vi "Dialog - Configure Packet Header.vi"(8 "error in (no error)":errorcluster, 9 "Header Elements In":bool[](array[boolean]), 11 "Packet Ref in":T1 format="%.0x") -> (0 "error out":errorcluster, 1 "Header Elements Out":bool[](array[boolean]), 3 "Packet Ref out":T1 format="%.0x")   [LabVIEW 2023, in "UDP-Custom-Device System Explorer.lvlib"]
uses:
  UDP-Custom-Device System Explorer.lvlib
  <vilib>/NI VeriStand/Custom Device API/Custom Device Item Ref.ctl
  <vilib>/NI VeriStand/Custom Device API/Custom Device API.lvlib
panel:
  in  "Source Node Name":bool
  in  "System Definition Version":bool
  in  "Protocol Revision":bool
  in  "Packet Size":bool=TRUE
  in  "TimeStamp":bool
  out "Data Header":string="Data"
  out "Num Bits Header":string="Num Bits"
  out "Data":string
  out "Num Bits":string
  in  "Cancel":bool
  in  "OK":bool
  in  "Packet Sequence":bool
  in  "Packet ID":bool
  in  "Num of Chans":bool
  # "Select Packet Header Information"
  # "Sample Packet Header"
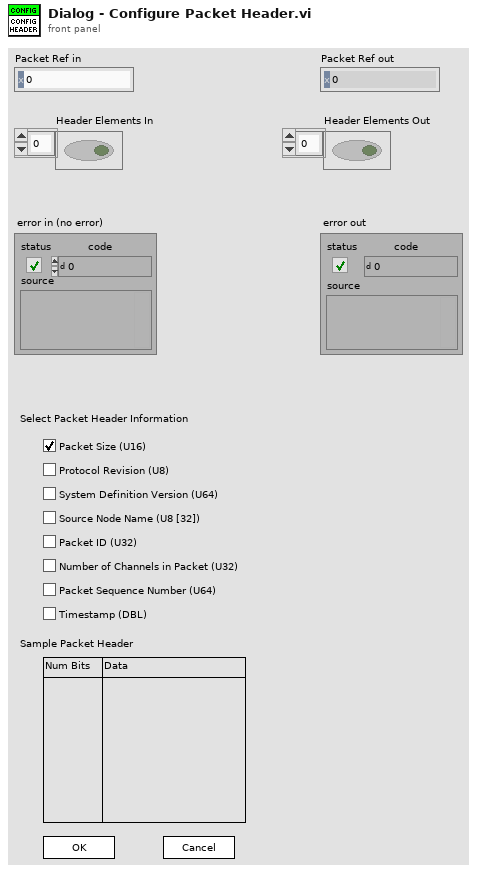
[diagram p1: front panel]
types:
  T1 = typedef "Custom Device API.lvlib/Custom Device Item Ref.ctl" = u64
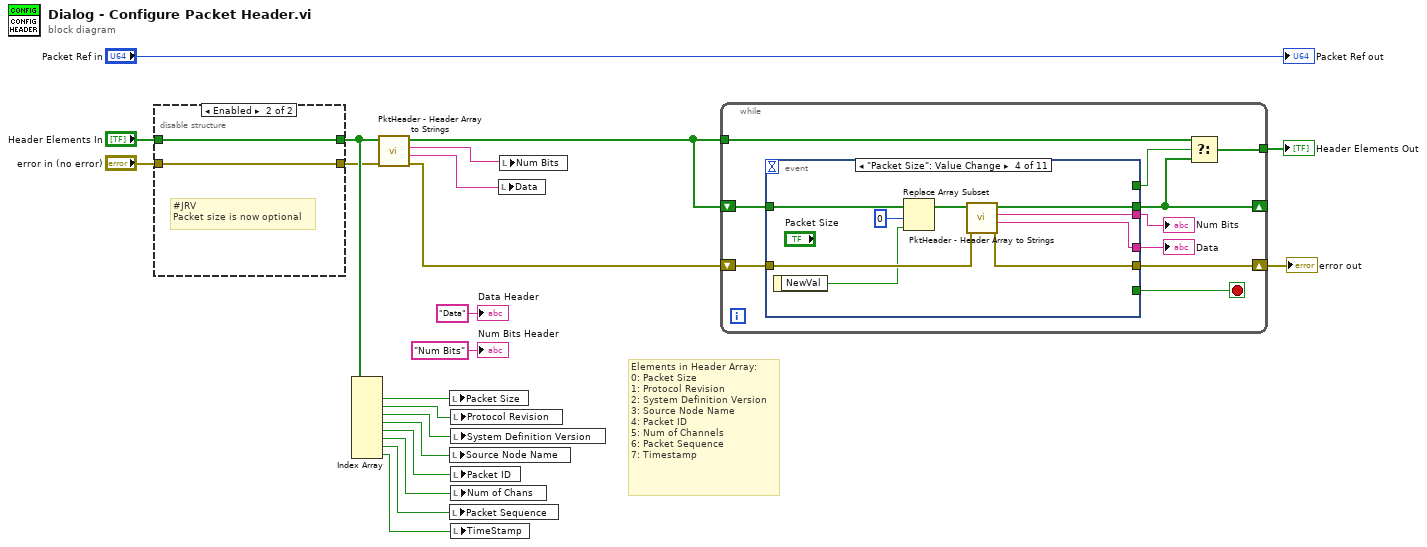
[diagram p0: block diagram]
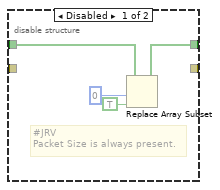
[diagram p2: hidden frame]
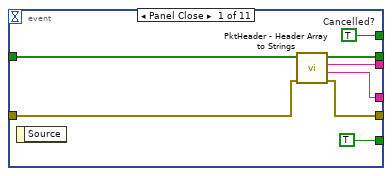
[diagram p3: hidden frame]
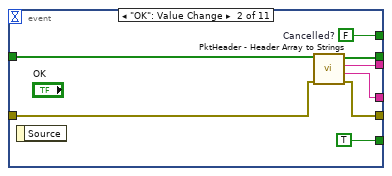
[diagram p4: hidden frame]
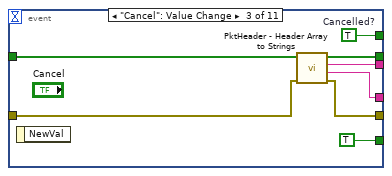
[diagram p5: hidden frame]
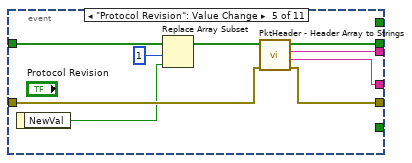
[diagram p6: hidden frame]
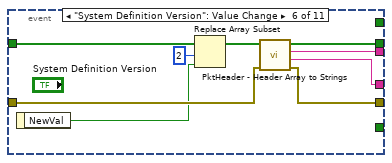
[diagram p7: hidden frame]
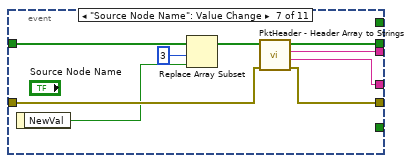
[diagram p8: hidden frame]
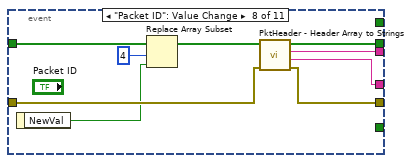
[diagram p9: hidden frame]
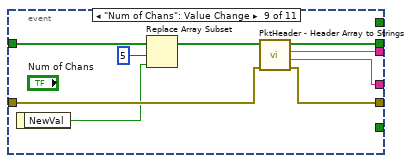
[diagram p10: hidden frame]
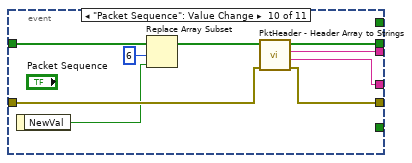
[diagram p11: hidden frame]
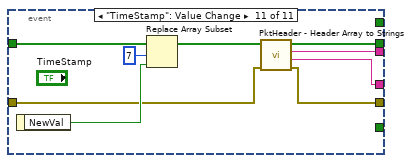
[diagram p12: hidden frame]
diagram:
  # "Elements in Header Array:\n0: Packet Size\n1: Protocol Revision\n2: System Definition Version\n3: Source Node Name\n4: Packet ID\n5: Num of Channels\n6: Packet Sequence\n7: Timestamp"
  n1 = disable-structure shown="Enabled" {
    disable-tunnel: "Header Elements In" -> [w24 w27]
    disable-tunnel: [w23 w27] -> w3
    disable-tunnel: [_ w26] -> w2
    disable-tunnel: "error in (no error)" -> [_ w26]
    frame Disabled {
      # "#JRV\nPacket Size is always present."
      n2 = Replace Array Subset(array=w24, new element=TRUE ("new element/subarray"), index=0) -> (w23:bool[])
    }
    frame Enabled {
      # "#JRV\nPacket size is now optional"
    }
  }
  n3 = Index Array(array=w3) -> (element #1=w12:bool, element #2=w11:bool, element #3=w10:bool, element #4=w9:bool, element #5=w8:bool, element #6=w7:bool, element #7=w6:bool, element #8=w5:bool)  [unwired: 8 in]
  n4 = call "PktHeader - Header Array to Strings.vi"("error in (no error)"=w2, "Header Array In"=w3) -> ("error out"=w13:errorcluster, "Data Name String"=w14:string, "Num Bits String"=w15:string, "Header Array Out"=w16:bool[])  [unwired: 6 in]
  n5 = local write "Packet Size"(w12) -> ()
  n6 = local write "Source Node Name"(w9) -> ()
  n7 = local write "Packet Sequence"(w6) -> ()
  n8 = local write "Protocol Revision"(w11) -> ()
  n9 = local write "System Definition Version"(w10) -> ()
  n10 = local write "Packet ID"(w8) -> ()
  n11 = local write "Num of Chans"(w7) -> ()
  n12 = local write "TimeStamp"(w5) -> ()
  n13 = local write "Data"(w14) -> ()
  n14 = local write "Num Bits"(w15) -> ()
  n15 = while {
    tunnel: w16 -> [w35]
    shift-right: [w32] -> _
    shift-left: w16 -> [w37]
    tunnel: [w34] -> w21
    shift-right: [w30] -> w17
    shift-left: w13 -> [w31]
    stop <- w36 stop-if-true
    n16 = event shown="[3] \"Packet Size\": Value Change" {
      selector: _ -> [_ _ _ _ _ _ _ _ _ _ _]
      dyn-events: _ -> [_ _ _ _ _ _ _ _ _ _ _]
      timeout: _ -> [_ _ _ _ _ _ _ _ _ _ _]
      tunnel: w37 -> [w43 w51 w59 w70 w79 w88 w97 w106 w115 w124 w133]
      tunnel: [w42 w50 w58 w67 w76 w85 w94 w103 w112 w121 w127] -> w32
      tunnel: [w45 w53 w61 _ _ _ _ _ _ _ _] -> w33
      tunnel: [TRUE TRUE TRUE _ _ _ _ _ _ _ _] -> w36
      tunnel: w31 -> [w38 w46 w54 w66 w75 w84 w93 w102 w111 w120 w129]
      tunnel: [w40 w48 w56 w65 w74 w83 w92 w101 w110 w119 w128] -> w30
      tunnel: [w41 w49 w57 w64 w73 w82 w91 w100 w109 w118 w126] -> w29
      tunnel: [w39 w47 w55 w63 w72 w81 w90 w99 w108 w117 w125] -> w28
      event Panel Close {
        w45 = TRUE  # Cancelled?
        n17 = event-data() -> ()  [unwired: 1 in, 1 out]
        n18 = call "PktHeader - Header Array to Strings.vi"("error in (no error)"=w38, "Header Array In"=w43) -> ("error out"=w40:errorcluster, "Data Name String"=w39:string, "Num Bits String"=w41:string, "Header Array Out"=w42:bool[])  [unwired: 6 in]
      }
      event "OK": Value Change {
        w53 = FALSE  # Cancelled?
        n19 = event-data() -> ()  [unwired: 1 in, 1 out]
        n20 = call "PktHeader - Header Array to Strings.vi"("error in (no error)"=w46, "Header Array In"=w51) -> ("error out"=w48:errorcluster, "Data Name String"=w47:string, "Num Bits String"=w49:string, "Header Array Out"=w50:bool[])  [unwired: 6 in]
      }
      event "Cancel": Value Change {
        w61 = TRUE  # Cancelled?
        n21 = event-data() -> ()  [unwired: 1 in, 1 out]
        n22 = call "PktHeader - Header Array to Strings.vi"("error in (no error)"=w54, "Header Array In"=w59) -> ("error out"=w56:errorcluster, "Data Name String"=w55:string, "Num Bits String"=w57:string, "Header Array Out"=w58:bool[])  [unwired: 6 in]
      }
      event "Packet Size": Value Change {
        n23 = event-data() -> ("NewVal"=w62:bool)  [unwired: 1 in]
        n24 = Replace Array Subset(array=w70, new element=w62, index=0) -> (w68:bool[])
        n25 = call "PktHeader - Header Array to Strings.vi"("error in (no error)"=w66, "Header Array In"=w68) -> ("error out"=w65:errorcluster, "Data Name String"=w63:string, "Num Bits String"=w64:string, "Header Array Out"=w67:bool[])  [unwired: 6 in]
      }
      event "Protocol Revision": Value Change {
        n26 = event-data() -> ("NewVal"=w71:bool)  [unwired: 1 in]
        n27 = Replace Array Subset(array=w79, new element=w71, index=1) -> (w77:bool[])
        n28 = call "PktHeader - Header Array to Strings.vi"("error in (no error)"=w75, "Header Array In"=w77) -> ("error out"=w74:errorcluster, "Data Name String"=w72:string, "Num Bits String"=w73:string, "Header Array Out"=w76:bool[])  [unwired: 6 in]
      }
      event "System Definition Version": Value Change {
        n29 = event-data() -> ("NewVal"=w80:bool)  [unwired: 1 in]
        n30 = Replace Array Subset(array=w88, new element=w80, index=2) -> (w86:bool[])
        n31 = call "PktHeader - Header Array to Strings.vi"("error in (no error)"=w84, "Header Array In"=w86) -> ("error out"=w83:errorcluster, "Data Name String"=w81:string, "Num Bits String"=w82:string, "Header Array Out"=w85:bool[])  [unwired: 6 in]
      }
      event "Source Node Name": Value Change {
        n32 = event-data() -> ("NewVal"=w89:bool)  [unwired: 1 in]
        n33 = Replace Array Subset(array=w97, new element=w89, index=3) -> (w95:bool[])
        n34 = call "PktHeader - Header Array to Strings.vi"("error in (no error)"=w93, "Header Array In"=w95) -> ("error out"=w92:errorcluster, "Data Name String"=w90:string, "Num Bits String"=w91:string, "Header Array Out"=w94:bool[])  [unwired: 6 in]
      }
      event "Packet ID": Value Change {
        n35 = event-data() -> ("NewVal"=w98:bool)  [unwired: 1 in]
        n36 = Replace Array Subset(array=w106, new element=w98, index=4) -> (w104:bool[])
        n37 = call "PktHeader - Header Array to Strings.vi"("error in (no error)"=w102, "Header Array In"=w104) -> ("error out"=w101:errorcluster, "Data Name String"=w99:string, "Num Bits String"=w100:string, "Header Array Out"=w103:bool[])  [unwired: 6 in]
      }
      event "Num of Chans": Value Change {
        n38 = event-data() -> ("NewVal"=w107:bool)  [unwired: 1 in]
        n39 = Replace Array Subset(array=w115, new element=w107, index=5) -> (w113:bool[])
        n40 = call "PktHeader - Header Array to Strings.vi"("error in (no error)"=w111, "Header Array In"=w113) -> ("error out"=w110:errorcluster, "Data Name String"=w108:string, "Num Bits String"=w109:string, "Header Array Out"=w112:bool[])  [unwired: 6 in]
      }
      event "Packet Sequence": Value Change {
        n41 = event-data() -> ("NewVal"=w116:bool)  [unwired: 1 in]
        n42 = Replace Array Subset(array=w124, new element=w116, index=6) -> (w122:bool[])
        n43 = call "PktHeader - Header Array to Strings.vi"("error in (no error)"=w120, "Header Array In"=w122) -> ("error out"=w119:errorcluster, "Data Name String"=w117:string, "Num Bits String"=w118:string, "Header Array Out"=w121:bool[])  [unwired: 6 in]
      }
      event "TimeStamp": Value Change {
        n44 = event-data() -> ("NewVal"=w131:bool)  [unwired: 1 in]
        n45 = Replace Array Subset(array=w133, new element=w131, index=7) -> (w130:bool[])
        n46 = call "PktHeader - Header Array to Strings.vi"("error in (no error)"=w129, "Header Array In"=w130) -> ("error out"=w128:errorcluster, "Data Name String"=w125:string, "Num Bits String"=w126:string, "Header Array Out"=w127:bool[])  [unwired: 6 in]
      }
    }
    "Num Bits" <- w29
    "Data" <- w28
    n47 = Select(t=w35, s=w33, f=w32) -> (s? t:f=w34:bool[])
  }
  "error out" <- w17
  "Header Elements Out" <- w21
  "Packet Ref out" <- "Packet Ref in"
  "Num Bits Header" <- "Num Bits" ("Num Bits Header")
  "Data Header" <- "Data" ("Data Header")
